vi "Load Virt Instrs.vi"(8 "error in":errorcluster, 10 "Local Virt Instrs":T1(array[cluster]), 11 "MSS in":refnum<class "MSS.lvclass">) -> (0 "error out":errorcluster, 3 "MSS out":refnum<class "MSS.lvclass">)   [LabVIEW 2023, in "HAL.lvlib" / "MSS.lvclass"]
uses:
  MSS.lvclass
  MSS.lvclass/MSS.ctl
  Virtual Instruments/Virtual Instrument/Virtual Instrument.lvclass
  Virtual Instruments/Perform Action Strategy/Perform Action Strategy.lvclass
  Virtual Instruments/Virtual Instrument/Virtual Instrument.lvclass/Virtual Instrument.ctl
  Virtual Instruments/Scaling Strategy/Scaling Strategy.lvclass
  Virtual Instruments/No Scaling/No Scaling.lvclass
  <vilib>/Utility/miscctls.llb/LVMapReplaceAction.ctl
  7ac0bb8c-1788-4fef-907a-541b59c50176.vi
  42e74922-bfaa-4b06-953c-15db6f3e949b.vi
  <vilib>/JDP Science/JSONtext/JSON text to Variant.vi
  <vilib>/JDP Science/JSONtext/LVClass Serializer/JSONtext LVClass Serializer.lvclass
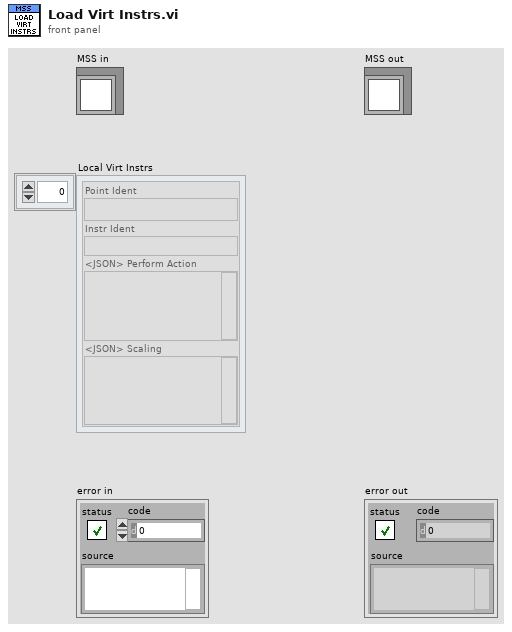
[diagram p1: front panel]
types:
  T1 = cluster{"Point Ident":string, "Instr Ident":string, "<JSON> Perform Action":string, "<JSON> Scaling":string}[]
  T2 = map{string, refnum<class "Virtual Instrument.lvclass">}
  T3 = map{string, cluster{"Instrument":refnum<class "Instrument.lvclass">, "Ref Count":i16}}
  T4 = cluster{"Class":string, "<JSON>Constants":string}
  T5 = typedef "LVMapReplaceAction.ctl" = enum32{"Modify Entry only if found", "Add or Modify Entry", "Delete Entry"}
  T6 = cluster{"Instrument":refnum<class "Instrument.lvclass">, "Ref Count":i16}
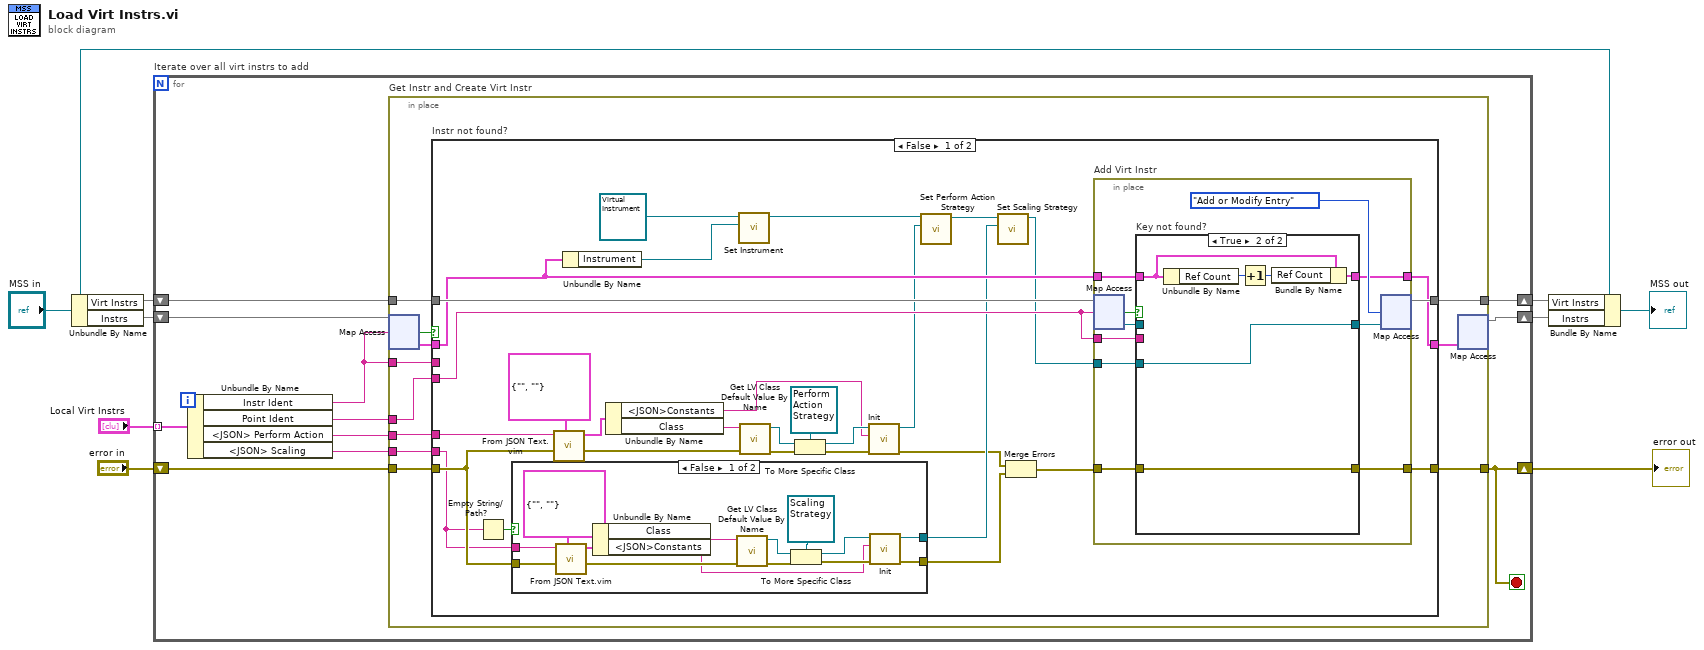
[diagram p0: block diagram]
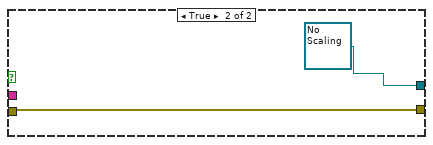
[diagram p2: hidden frame]
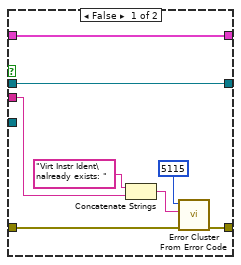
[diagram p3: hidden frame]
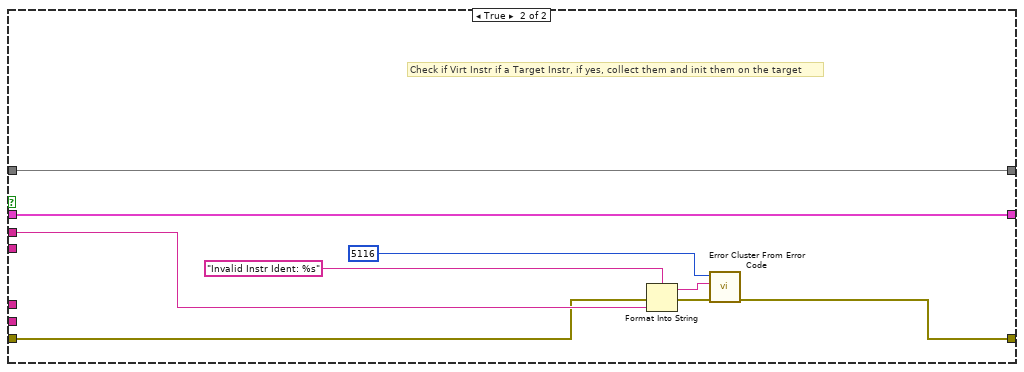
[diagram p4: hidden frame]
diagram:
  n1 = Unbundle By Name("MSS in") -> ("Virt Instrs"=w5:T2, "Instrs"=w6:T3)
  n2 = for "Iterate over all virt instrs to add" {
    tunnel: "Local Virt Instrs" -> [w14] mode=indexing
    shift-right: [w17] -> w8
    shift-left: "error in" -> [w19]
    shift-right: [w11] -> w3
    shift-left: w6 -> [w15]
    shift-right: [w12] -> w4
    shift-left: w5 -> [w13]
    stop <- w17 stop-if-true
    n3 = Unbundle By Name(w14) -> ("Instr Ident"=w10:string, "Point Ident"=w16:string, "<JSON> Perform Action"=w18:string, "<JSON> Scaling"=w20:string)
    n4 = in-place "Get Instr and Create Virt Instr" {
      in-place-border: w20 -> [w31]
      in-place-border: w19 -> [w30]
      in-place-border: w18 -> [w29]
      in-place-border: [w28] -> w17
      in-place-border: w16 -> [w27]
      in-place-border: w10 -> [w21]
      in-place-border: w13 -> [w23]
      in-place-border: [w22] -> w12
      n5 = in-place-map #1(w15, w10) -> (w26:T6, w24:bool)  [unwired: 1 in]
      n6 = case "Instr not found?" shown="False" w24 {
        tunnel: w31 -> [w35 _]
        tunnel: w30 -> [w43 w106]
        tunnel: w29 -> [w59 _]
        tunnel: [w57 w110] -> w28
        tunnel: w27 -> [w53 _]
        tunnel: w23 -> [w55 w108]
        tunnel: [w58 w108] -> w22
        tunnel: w26 -> [w47 w109]
        tunnel: [w56 w109] -> w25
        tunnel: w21 -> [_ w107]
        frame False {
          n7 = Empty String/Path?(string/path=w35) -> (empty?=w36:bool)
          n8 = case shown="False" w36 {
            tunnel: w35 -> [w74 _]
            tunnel: w43 -> [w73 w76]
            tunnel: [w65 refnum<class "No Scaling.lvclass"> refnum ("HAL.lvlib:No Scaling.lvclass")] -> w39
            tunnel: [w62 w76] -> w38
            frame False {
              n9 = call "From JSON Text.vim"("Data Type and Default Value"=T4 {"Class"="", "<JSON>Constants"=""}, "error in (no error)"=w73, "JSON"=w74) -> ("error out"=w70:errorcluster, "Data out"=w72:T4)  [unwired: 7 in]
              n10 = Unbundle By Name(w72) -> ("Class"=w71:string, "<JSON>Constants"=w63:string)
              n11 = call <vilib>:"Get LV Class Default Value By Name.vi"("error in (no error)"=w70, "class name"=w71) -> ("error out"=w68:errorcluster, "object"=w69:refnum<class>)  [unwired: 8 in]
              n12 = To More Specific Class(target class=refnum<class "Scaling Strategy.lvclass"> refnum ("HAL.lvlib:Scaling Strategy.lvclass"), reference=w69, error in=w68) -> (specific class reference=w66:refnum<class "Scaling Strategy.lvclass">, error out=w64:errorcluster)
              n13 = call-dynamic "Init.vi"("error in"=w64, "<JSON> Scaling Data"=w63, "Scaling Strategy in"=w66) -> ("error out"=w62:errorcluster, "Scaling Strategy out"=w65:refnum<class "Scaling Strategy.lvclass">)  [unwired: 7 in]
            }
            frame True {
            }
          }
          n14 = call "From JSON Text.vim"("Data Type and Default Value"=T4 {"Class"="", "<JSON>Constants"=""}, "error in (no error)"=w43, "JSON"=w59) -> ("error out"=w50:errorcluster, "Data out"=w49:T4)  [unwired: 7 in]
          n15 = Unbundle By Name(w47) -> ("Instrument"=w45:refnum<class "Instrument.lvclass">)
          n16 = Unbundle By Name(w49) -> ("<JSON>Constants"=w40:string, "Class"=w48:string)
          n17 = call "Set Instrument.vi"("HAL.lvlib:Instrument"=w45, "Virtual Instrument in"=refnum<class "Virtual Instrument.lvclass"> refnum ("HAL.lvlib:Virtual Instrument.lvclass")) -> ("Virtual Instrument out"=w44:refnum<class "Virtual Instrument.lvclass">)  [unwired: 9 in]
          n18 = call <vilib>:"Get LV Class Default Value By Name.vi"("error in (no error)"=w50, "class name"=w48) -> ("error out"=w61:errorcluster, "object"=w60:refnum<class>)  [unwired: 8 in]
          n19 = To More Specific Class(target class=refnum<class "Perform Action Strategy.lvclass"> refnum ("HAL.lvlib:Perform Action Strategy.lvclass"), reference=w60, error in=w61) -> (specific class reference=w41:refnum<class "Perform Action Strategy.lvclass">, error out=w54:errorcluster)
          n20 = call-dynamic "Init.vi"("error in"=w54, "<JSON> Const Action Data"=w40, "Perform Action Strategy in"=w41) -> ("error out"=w34:errorcluster, "Perform Action Strategy out"=w33:refnum<class "Perform Action Strategy.lvclass">)  [unwired: 7 in]
          n21 = call "Set Perform Action Strategy.vi"("Perform Action Strategy"=w33, "Action Performer in"=w44) -> ("Action Performer out"=w32:refnum<class "Virtual Instrument.lvclass">)  [unwired: 9 in]
          n22 = call "Set Scaling Strategy.vi"("Scaling Strategy"=w39, "Virtual Instrument in"=w32) -> ("Virtual Instrument out"=w37:refnum<class "Virtual Instrument.lvclass">)  [unwired: 9 in]
          n23 = Merge Errors(w34, w38) -> (w42:errorcluster)
          n24 = in-place "Add Virt Instr" {
            in-place-border: w42 -> [w85]
            in-place-border: [w84] -> w57
            in-place-border: [w82] -> w56
            in-place-border: w47 -> [w81]
            in-place-border: w53 -> [w80]
            in-place-border: w37 -> [w79]
            n25 = in-place-map #2(w55, w53) -> (w86:refnum<class "Virtual Instrument.lvclass">, w87:bool)  [unwired: 1 in]
            n26 = case "Key not found?" shown="True" w87 {
              tunnel: w86 -> [w94 _]
              tunnel: [w94 w96] -> w78
              tunnel: w85 -> [w95 w101]
              tunnel: [w92 w101] -> w84
              tunnel: w81 -> [w93 w98]
              tunnel: [w93 w97] -> w82
              tunnel: w80 -> [w88 _]
              tunnel: w79 -> [_ w96]
              frame False {
                n27 = Concatenate Strings("Virt Instr Ident\nalready exists: " ("string"), w88) -> (w90:string)
                n28 = call <vilib>:"Error Cluster From Error Code.vi"("error in (no error)"=w95, "error message (\"\")"=w90, "error code (0)"=5115) -> ("error out"=w92:errorcluster)  [unwired: 6 in]
              }
              frame True {
                n29 = Unbundle By Name(w98) -> ("Ref Count"=w100:i16)
                n30 = Increment(x=w100) -> (x+1=w99:i16)
                n31 = Bundle By Name(cluster=w98, "Ref Count"=w99) -> (w97:T6)
              }
            }
            n32 = in-place-map #2(w78, LVMapReplaceAction."Add or Modify Entry" ("action")) -> (w58:T2)  [unwired: 2 out]
          }
        }
        frame True {
          # "Check if Virt Instr if a Target Instr, if yes, collect them and init them on the target"
          n33 = Format Into String(format string="Invalid Instr Ident: %s" ("string"), error in=w106, w107) -> (resulting string=w102:string, error out=w104:errorcluster)  [unwired: 1 in]
          n34 = call <vilib>:"Error Cluster From Error Code.vi"("error in (no error)"=w104, "error message (\"\")"=w102, "error code (0)"=5116) -> ("error out"=w110:errorcluster)  [unwired: 6 in]
        }
      }
      n35 = in-place-map #1(w25) -> (w11:T3)  [unwired: 1 in, 2 out]
    }
  }
  "error out" <- w8
  n36 = Bundle By Name(cluster="MSS in", "Virt Instrs"=w4, "Instrs"=w3) -> (→"MSS out":refnum<class "MSS.lvclass">)
